vi "gfitsio-get-column-number.vi"(6 "case sensitive? (F:No)":bool, 7 "column":string, 8 "error in (no error)":errorcluster, 11 "gfits refnum":T1) -> (0 "error out":errorcluster, 2 "colnum":i32, 3 "dup gfits refnum":T1)   [LabVIEW 2014, in "gfitsio.lvlib"]
doc: "Get the table column number of the column whose name matches an input template name. As a general rule, the column names should be treated as case INsensitive.\n\nThe input column name template may be either the exact name of the column to be searched for, or it may contain wild card characters (*, ?, or #), or it may contain the integer number of the desired column (with the first column = 1). The `*' wild card character matches any sequence of characters (including zero characters) and the `?' character matches any single character. The # wildcard will match any consecutive string of decimal digits (0-9). If more than one column name in the table matches the template string, then the first match is returned.\n\nThe FITS Standard recommends that only letters, digits, and the underscore character be used in column names (with no embedded spaces). Trailing blank characters are not significant. It is recommended that all the column names in a given table be unique within the first 8 characters, and strongly recommended that the names be unique within the first 16 characters."
uses:
  gfitsio.lvlib
  gfitsio-refnum.ctl
  gfitsio.dll
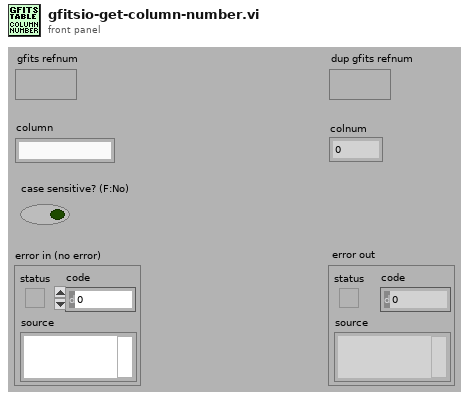
[diagram p1: front panel]
types:
  T1 = typedef "gfitsio.lvlib/gfitsio-refnum.ctl" = refnum<k1>
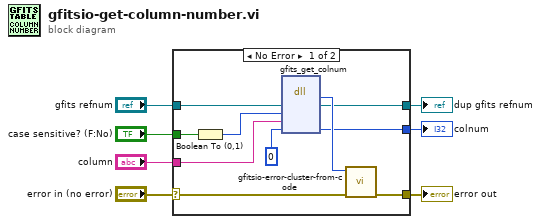
[diagram p0: block diagram]
diagram:
  n1 = case shown="No Error" "error in (no error)" {
    selector: "error in (no error)" -> [w16 w19]
    tunnel: [w15 w19] -> w7
    tunnel: "gfits refnum" -> [w13 w18]
    tunnel: [w14 w18] -> w5
    tunnel: [w8 _] -> w3
    tunnel: "column" -> [w10 _]
    tunnel: "case sensitive? (F:No)" -> [w12 _]
    frame No Error {
      n2 = Boolean To (0,1)(Boolean=w12) -> (0, 1=w11:i16)
      n3 = dll-call lib="D:/optics_and_proj_related_stuff/labview_codes/gfitsio/gfitsio.dll" fn="gfits_get_colnum"("gfits refnum"=w13, "casesen"=w11, "column"=w10, "colnum"=0) -> (w17:i32, "gfits refnum"=w14:T1, "colnum"=w8:i32)  [unwired: 4 in, 3 out]
      n4 = call "gfitsio-error-cluster-from-code.vi"("error in (no error)"=w16, "error code"=w17) -> ("error out"=w15:errorcluster)  [unwired: 9 out]
    }
    frame Error {
    }
  }
  "error out" <- w7
  "dup gfits refnum" <- w5
  "colnum" <- w3
